vi "Store Data.vi"(5 "MeasurementNumber":i32 format="%.0g", 6 "DataFormat":string, 7 "TraceType":string, 8 "error in (no error)":errorcluster {"code" format="%.0x"}, 9 "TypeData":string, 10 "FileName":string, 11 "instrument handle":refnum<k15>) -> (0 "error out":errorcluster {"code" format="%.0x"}, 3 "instrument handle out":refnum<k15>)   [LabVIEW 2014, in "Agilent NA.lvlib"]
doc: "Stores trace data to the following file types: *.prn, *.cti, *.csv, *.mdf"
uses:
  Agilent NA.lvlib
  AgNA.dll
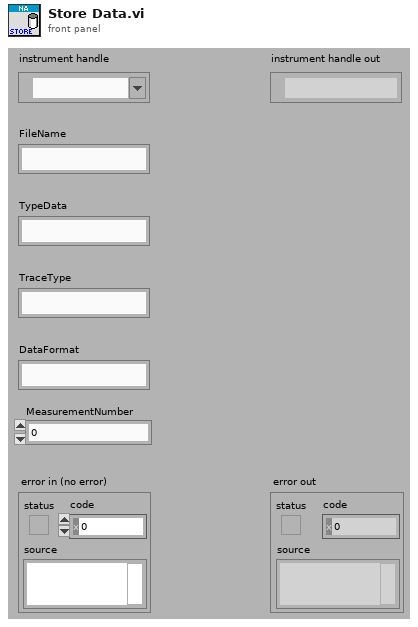
[diagram p1: front panel]
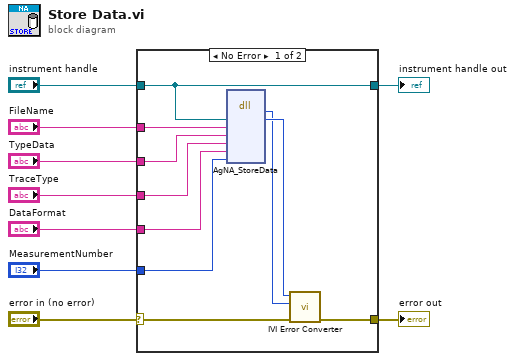
[diagram p0: block diagram]
diagram:
  n1 = case shown="No Error" "error in (no error)" {
    selector: "error in (no error)" -> [w17 w21]
    tunnel: [w16 w21] -> w9
    tunnel: "FileName" -> [w15 _]
    tunnel: "TypeData" -> [w14 _]
    tunnel: "TraceType" -> [w13 _]
    tunnel: "DataFormat" -> [w12 _]
    tunnel: "MeasurementNumber" -> [w11 _]
    tunnel: [w10 w20] -> w2
    tunnel: "instrument handle" -> [w10 w20]
    frame No Error {
      n2 = dll-call lib="AgNA**.dll" fn="AgNA_StoreData"("Vi"=w10, "FileName"=w15, "TypeData"=w14, "TraceType"=w13, "DataFormat"=w12, "MeasurementNumber"=w11) -> (w18:i32, "Vi"=w19:u32)  [unwired: 8 in, 2 out]
      n3 = call "IVI Error Converter.vi"("error in (no error)"=w17, "IVI error code (0)"=w18, "instrument handle"=w19) -> ("error out"=w16:errorcluster)  [unwired: 7 in, 1 out]
    }
    frame Error {
    }
  }
  "error out" <- w9
  "instrument handle out" <- w2
